vi "clusterTOinput.vi"(5 "Set_Rel":T2 {"Numeric" format="%#_4f"}, 11 "error in (no error)":errorcluster) -> (6 "Range":T4, 8 "Numeric":i32, 10 "Unit":T3, 15 "error out":errorcluster)   [LabVIEW 2014, in "FH 55.lvlib"]
uses:
  FH 55.lvlib
  TypeDef/Range.ctl
  TypeDef/Unit.ctl
  TypeDef/Unit2.ctl
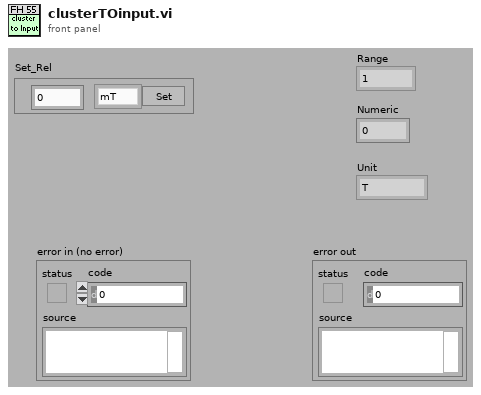
[diagram p1: front panel]
types:
  T1 = typedef "FH 55.lvlib/Unit2.ctl" = enum16{"mT", "G", "kA/m"}
  T2 = cluster{"Numeric":dbl, "Cancel Button":bool, "Unit":T1}
  T3 = typedef "FH 55.lvlib/Unit.ctl" = enum16{"T", "G", "A/m"}
  T4 = typedef "FH 55.lvlib/Range.ctl" = enum16{"1", "2", "3", "4", "5", "6", "7"}
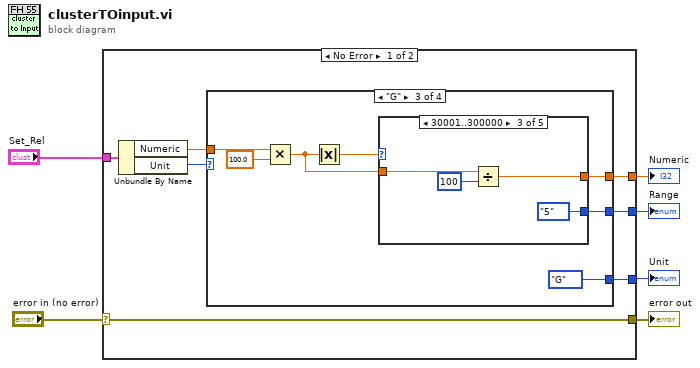
[diagram p0: block diagram]
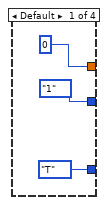
[diagram p2: hidden frame]
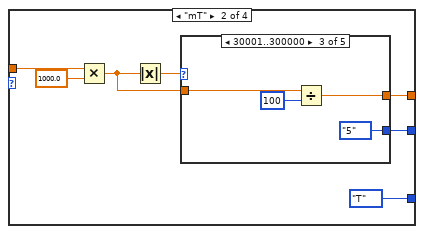
[diagram p3: hidden frame]
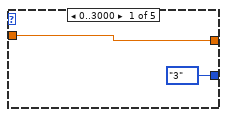
[diagram p4: hidden frame]
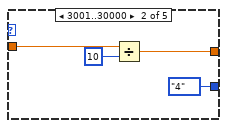
[diagram p5: hidden frame]
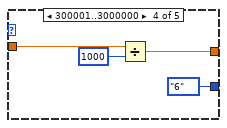
[diagram p6: hidden frame]
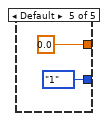
[diagram p7: hidden frame]
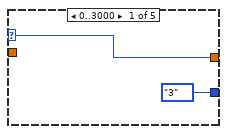
[diagram p8: hidden frame]
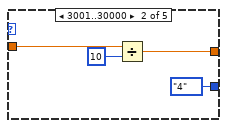
[diagram p9: hidden frame]
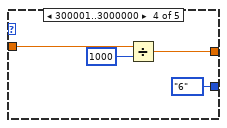
[diagram p10: hidden frame]
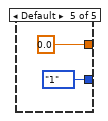
[diagram p11: hidden frame]
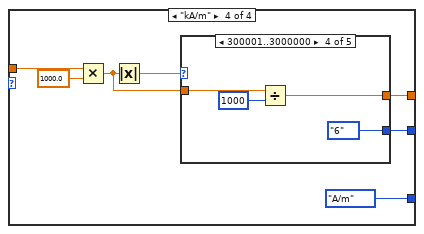
[diagram p12: hidden frame]
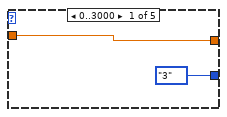
[diagram p13: hidden frame]
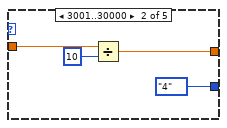
[diagram p14: hidden frame]
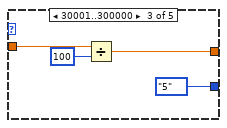
[diagram p15: hidden frame]
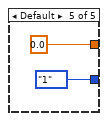
[diagram p16: hidden frame]
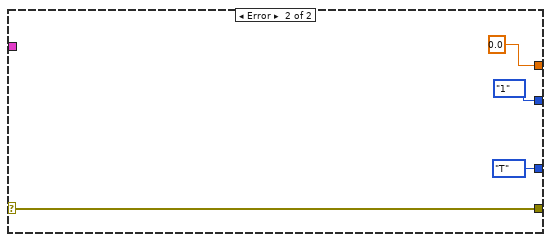
[diagram p17: hidden frame]
diagram:
  n1 = case shown="No Error" "error in (no error)" {
    selector: "error in (no error)" -> [w8 w89]
    tunnel: "Set_Rel" -> [w13 _]
    tunnel: [w8 w89] -> w5
    tunnel: [w10 Unit."T" ("Unit")] -> w4
    tunnel: [w9 Range."1" ("Range")] -> w3
    tunnel: [w7 0.0] -> w2
    frame No Error {
      n2 = Unbundle By Name(w13) -> ("Numeric"=w12:dbl, "Unit"=w11:T1)
      n3 = case shown="\"G\"" w11 {
        tunnel: w12 -> [_ w19 w42 w64]
        tunnel: [Unit."T" ("Unit") Unit."T" ("Unit") Unit."G" ("Unit") Unit."A/m" ("Unit")] -> w10
        tunnel: [Range."1" ("Range") w22 w45 w69] -> w9
        tunnel: [i64 0 ("Numeric") w20 w43 w67] -> w7
        frame Default {
        }
        frame "mT" {
          n4 = Multiply(x=w19, y=1000.0) -> (x*y=w17:dbl)
          n5 = Absolute Value(x=w17) -> (abs(x)=w18:dbl)
          n6 = case shown="30001..300000" w18 {
            tunnel: [Range."3" ("Range") Range."4" ("Range") Range."5" ("Range") Range."6" ("Range") Range."1" ("Range")] -> w22
            tunnel: [w24 w27 w31 w35 0.0] -> w20
            tunnel: w17 -> [w24 w26 w30 w34 _]
            frame 0..3000 {
            }
            frame 3001..30000 {
              n7 = Divide(x=w26, y=10) -> (x/y=w27:dbl)
            }
            frame 30001..300000 {
              n8 = Divide(x=w30, y=100) -> (x/y=w31:dbl)
            }
            frame 300001..3000000 {
              n9 = Divide(x=w34, y=1000) -> (x/y=w35:dbl)
            }
            frame Default {
            }
          }
        }
        frame "G" {
          n10 = Multiply(x=w42, y=100.0) -> (x*y=w40:dbl)
          n11 = Absolute Value(x=w40) -> (abs(x)=w41:dbl)
          n12 = case shown="30001..300000" w41 {
            selector: w41 -> [w48 _ _ _ _]
            tunnel: [Range."3" ("Range") Range."4" ("Range") Range."5" ("Range") Range."6" ("Range") Range."1" ("Range")] -> w45
            tunnel: [w48 w50 w54 w58 0.0] -> w43
            tunnel: w40 -> [_ w49 w53 w57 _]
            frame 0..3000 {
            }
            frame 3001..30000 {
              n13 = Divide(x=w49, y=10) -> (x/y=w50:dbl)
            }
            frame 30001..300000 {
              n14 = Divide(x=w53, y=100) -> (x/y=w54:dbl)
            }
            frame 300001..3000000 {
              n15 = Divide(x=w57, y=1000) -> (x/y=w58:dbl)
            }
            frame Default {
            }
          }
        }
        frame "kA/m" {
          n16 = Multiply(x=w64, y=1000.0) -> (x*y=w63:dbl)
          n17 = Absolute Value(x=w63) -> (abs(x)=w66:dbl)
          n18 = case shown="300001..3000000" w66 {
            tunnel: [Range."3" ("Range") Range."4" ("Range") Range."5" ("Range") Range."6" ("Range") Range."1" ("Range")] -> w69
            tunnel: [w70 w73 w77 w81 0.0] -> w67
            tunnel: w63 -> [w70 w72 w76 w80 _]
            frame 0..3000 {
            }
            frame 3001..30000 {
              n19 = Divide(x=w72, y=10) -> (x/y=w73:dbl)
            }
            frame 30001..300000 {
              n20 = Divide(x=w76, y=100) -> (x/y=w77:dbl)
            }
            frame 300001..3000000 {
              n21 = Divide(x=w80, y=1000) -> (x/y=w81:dbl)
            }
            frame Default {
            }
          }
        }
      }
    }
    frame Error {
    }
  }
  "error out" <- w5
  "Range" <- w3
  "Numeric" <- w2
  "Unit" <- w4
